vi "PSD3.vi"(8 "error in (no error)":errorcluster, 9 "axis":string, 10 "data":dbl[](array[numeric]), 11 "Refnum in":refnum<k35>) -> (0 "error out":errorcluster, 1 "parameters":dbl[](array[numeric]), 2 "Array":cluster{dbl, dbl, dbl[]}[](array[cluster]), 3 "Refnum out":refnum<k35>)   [LabVIEW 2019]
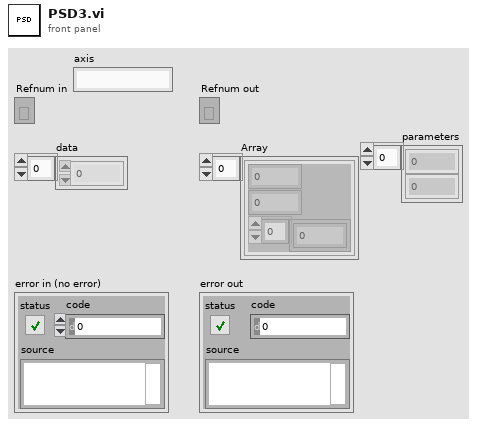
[diagram p1: front panel]
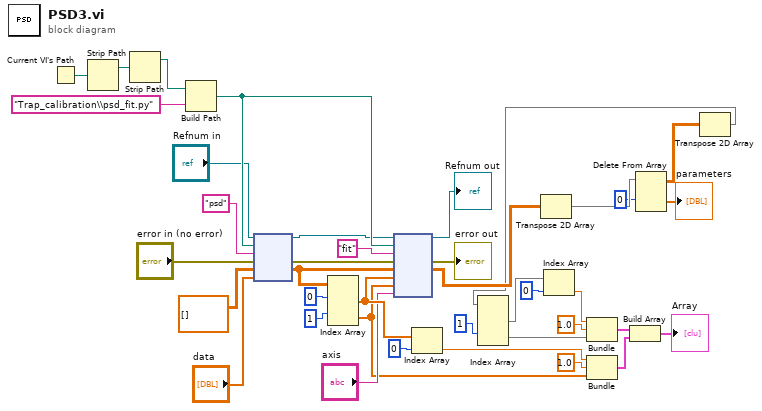
[diagram p0: block diagram]
diagram:
  n1 = Current VI's Path() -> (path=w14:path)
  n2 = Strip Path(path=w14) -> (stripped path=w8:path)  [unwired: 1 out]
  n3 = Strip Path(path=w8) -> (stripped path=w7:path)  [unwired: 1 out]
  n4 = Build Path(base path=w7, name or relative path="Trap_calibration\\psd_fit.py") -> (appended path=w21:path)
  n5 = node("Refnum in", w21, "psd" ("function name"), "error in (no error)", dbl[][] [], "data") -> (w17:refnum<k35>, w19:errorcluster, w22:dbl[][])  [unwired: 1 in, 2 out]
  n6 = Index Array(array=w22, index (row) #1=0 ("index (row)"), index (row) #2=1 ("index (row)")) -> (element #1=w28:dbl[], element #2=w23:dbl[])  [unwired: 2 in]
  n7 = node(w17, w21, "fit" ("function name"), w19, w22, w28, w23, "axis") -> (→"Refnum out":refnum<k35>, →"error out":errorcluster, w6:dbl[][])  [unwired: 3 in, 2 out]
  n8 = Index Array(array=w28, index=0) -> (element=w30:dbl)
  n9 = Transpose 2D Array(2D array=w6) -> (transposed array=w5:dbl[][])
  n10 = Bundle(w30, 1.0, w23) -> (w38:cluster{dbl, dbl, dbl[]})  [unwired: 1 in]
  n11 = Delete From Array(array=w5, index (row)=0) -> (deleted portion=→"parameters":dbl[], array with subset deleted=w2:dbl[][])  [unwired: 2 in]
  n12 = Transpose 2D Array(2D array=w2) -> (transposed array=w1:dbl[][])
  n13 = Index Array(array=w1, index (row) #2=1 ("index (row)")) -> (element #1=w31:dbl[], element #2=w26:dbl[])  [unwired: 3 in]
  n14 = Index Array(array=w31, index=0) -> (element=w34:dbl)
  n15 = Bundle(w34, 1.0, w26) -> (w37:cluster{dbl, dbl, dbl[]})  [unwired: 1 in]
  n16 = Build Array(w37, w38) -> (→"Array":cluster{dbl, dbl, dbl[]}[])
